vi "Query Instrument Information.vi"(0 "VISA resource name":refnum<visa-resource-name>, 11 "error in (no error)":errorcluster) -> (3 "Attenuator Cycle":string, 4 "VISA resource name out":refnum<visa-resource-name>, 6 "Power-On Cycle":string, 8 "Display-On Time":string, 10 "Option":string, 13 "Firmware Date":timestamp, 14 "Instrument-On Time":string, 15 "error out":errorcluster)   [LabVIEW 2011, in "Agilent PSG MXG Series.lvlib"]
doc: "Queries the diagnostic information of the signal generator.\n\n<B>Notes:</B>\n(1) For E8257D, E8267D, this VI is valid only when the instrument installs <B>Option 1E1</B> (Attenuator)."
uses:
  Agilent PSG MXG Series.lvlib
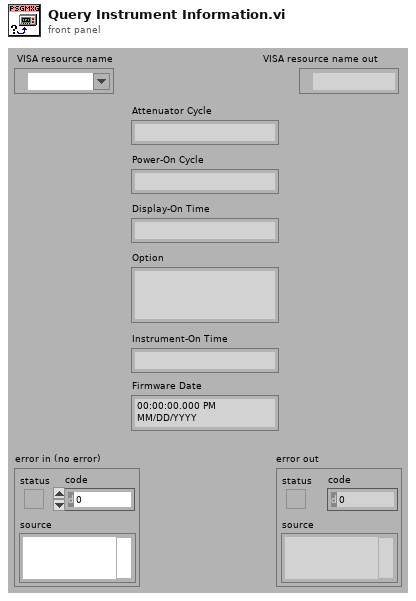
[diagram p1: front panel]
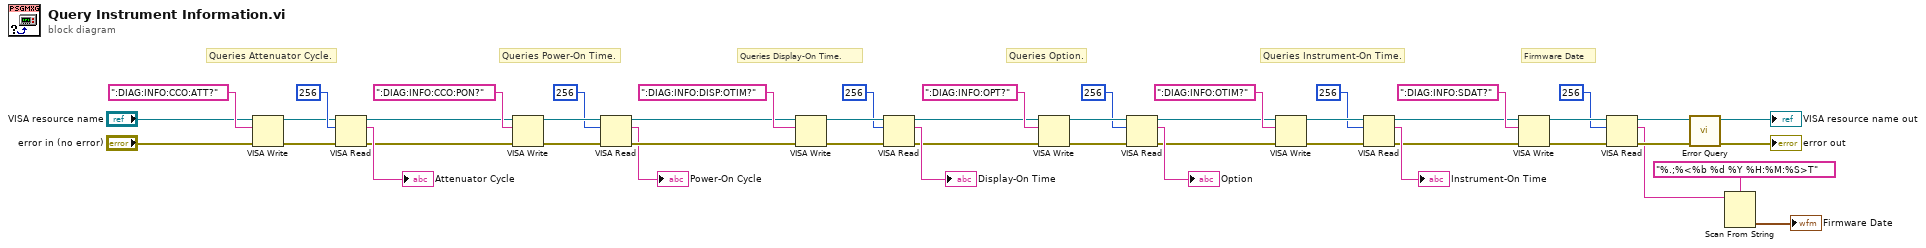
[diagram p0: block diagram]
diagram:
  # "Firmware Date"
  # "Queries Instrument-On Time."
  # "Queries Option."
  # "Queries Display-On Time."
  # "Queries Power-On Time."
  # "Queries Attenuator Cycle."
  n1 = VISA Write(VISA resource name="VISA resource name", write buffer=":DIAG:INFO:CCO:ATT?", error in (no error)="error in (no error)") -> (VISA resource name out=w46:refnum<visa-resource-name>, error out=w45:errorcluster)  [unwired: 1 out]
  n2 = VISA Read(VISA resource name=w46, byte count=u32 256, error in (no error)=w45) -> (VISA resource name out=w37:refnum<visa-resource-name>, read buffer=→"Attenuator Cycle":string, error out=w36:errorcluster)  [unwired: 1 out]
  n3 = VISA Write(VISA resource name=w37, write buffer=":DIAG:INFO:CCO:PON?", error in (no error)=w36) -> (VISA resource name out=w35:refnum<visa-resource-name>, error out=w34:errorcluster)  [unwired: 1 out]
  n4 = VISA Read(VISA resource name=w35, byte count=u32 256, error in (no error)=w34) -> (VISA resource name out=w32:refnum<visa-resource-name>, read buffer=→"Power-On Cycle":string, error out=w31:errorcluster)  [unwired: 1 out]
  n5 = VISA Write(VISA resource name=w32, write buffer=":DIAG:INFO:DISP:OTIM?", error in (no error)=w31) -> (VISA resource name out=w42:refnum<visa-resource-name>, error out=w41:errorcluster)  [unwired: 1 out]
  n6 = VISA Read(VISA resource name=w42, byte count=u32 256, error in (no error)=w41) -> (VISA resource name out=w28:refnum<visa-resource-name>, read buffer=→"Display-On Time":string, error out=w27:errorcluster)  [unwired: 1 out]
  n7 = VISA Write(VISA resource name=w28, write buffer=":DIAG:INFO:OPT?", error in (no error)=w27) -> (VISA resource name out=w26:refnum<visa-resource-name>, error out=w25:errorcluster)  [unwired: 1 out]
  n8 = VISA Read(VISA resource name=w26, byte count=u32 256, error in (no error)=w25) -> (VISA resource name out=w21:refnum<visa-resource-name>, read buffer=→"Option":string, error out=w20:errorcluster)  [unwired: 1 out]
  n9 = VISA Write(VISA resource name=w21, write buffer=":DIAG:INFO:OTIM?", error in (no error)=w20) -> (VISA resource name out=w19:refnum<visa-resource-name>, error out=w18:errorcluster)  [unwired: 1 out]
  n10 = VISA Read(VISA resource name=w19, byte count=u32 256, error in (no error)=w18) -> (VISA resource name out=w11:refnum<visa-resource-name>, read buffer=→"Instrument-On Time":string, error out=w10:errorcluster)  [unwired: 1 out]
  n11 = VISA Write(VISA resource name=w11, write buffer=":DIAG:INFO:SDAT?", error in (no error)=w10) -> (VISA resource name out=w14:refnum<visa-resource-name>, error out=w13:errorcluster)  [unwired: 1 out]
  n12 = VISA Read(VISA resource name=w14, byte count=u32 256, error in (no error)=w13) -> (VISA resource name out=w5:refnum<visa-resource-name>, read buffer=w3:string, error out=w4:errorcluster)  [unwired: 1 out]
  n13 = call "Error Query.vi"("error in (no error)"=w4, "VISA resource name"=w5) -> ("error out"=→"error out":errorcluster, "VISA resource name out"=→"VISA resource name out":refnum<visa-resource-name>)  [unwired: 6 in, 2 out]
  n14 = Scan From String(format string="%.;%<%b %d %Y %H:%M:%S>T", input string=w3) -> (output 1=→"Firmware Date":timestamp)  [unwired: 3 in, 3 out]
